vi "Write Skipped RUNs.vi"(8 "error in (no error)":errorcluster, 10 "Skipped RUNs":refnum<class "Schedule.lvclass">, 11 "Run Block in":refnum<class "Run Block.lvclass">) -> (0 "error out":errorcluster, 3 "Run Block out":refnum<class "Run Block.lvclass">)   [LabVIEW 2020, in "CIRCUS_uServices.lvlib" / "Run Utilities.lvlib" / "Run Block.lvclass"]
uses:
  Run Block.lvclass
  Schedule/Schedule.lvclass
  Run Block.lvclass/Run Block.ctl
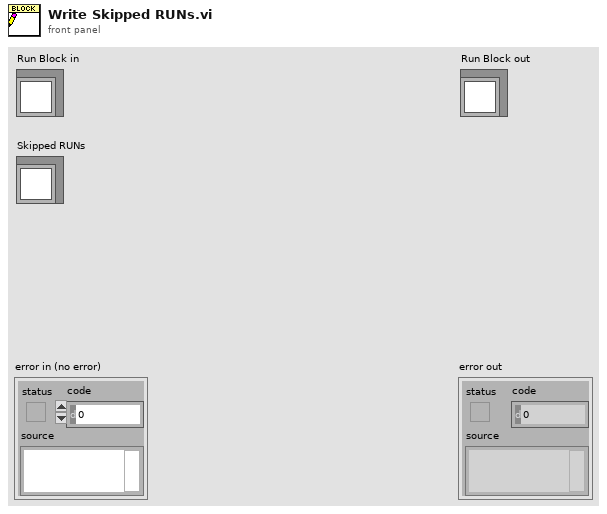
[diagram p1: front panel]
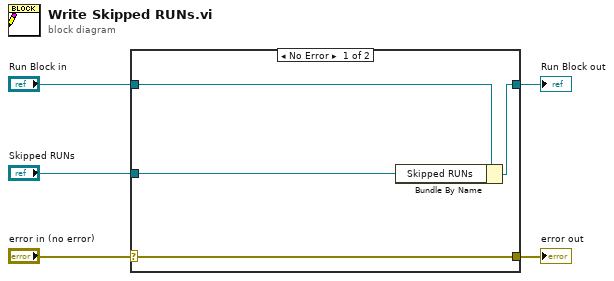
[diagram p0: block diagram]
diagram:
  n1 = case shown="No Error" "error in (no error)" {
    selector: "error in (no error)" -> [w9 w10]
    tunnel: [w9 w10] -> w4
    tunnel: [w7 w11] -> w2
    tunnel: "Run Block in" -> [w8 w11]
    tunnel: "Skipped RUNs" -> [w6 _]
    frame No Error {
      n2 = Bundle By Name(cluster=w8, "Skipped RUNs"=w6) -> (w7:refnum<class "Run Block.lvclass">)
    }
    frame Error {
    }
  }
  "error out" <- w4
  "Run Block out" <- w2
